vi "Target3.vi"() -> ()   [LabVIEW 2025]
uses:
  <vilib>/Platform/TimedLoop/XDataNode/timing_clust.ctl
  <vilib>/Platform/TimedLoop/XDataNode/nitl_modes.ctl
  <vilib>/Platform/TimedLoop/XDataNode/wakeup.ctl
  <vilib>/eio/utilities/niEioResolveVilibRelativePath.vi
  <vilib>/rvi/interface/RandomDataEmulation/niFpgaRandomDataHandleErrors.vi
  <vilib>/rvi/Emulation/niFpgaSctlEmulationGetInTimedLoop.vi
  <vilib>/rvi/Emulation/niFpgaEmulationReportErrorSimple.vi
  <vilib>/rvi/Emulation/niFpgaGetClockAttributes.vi
  <vilib>/rvi/Emulation/niFpgaCriticalErrorInLSC.vi
  <vilib>/rvi/linearAlgebra/MatrixMultiply/simVIs/SubVI/nifxpla_MatrixMultiply_SimMatrixSizes.vi
  <vilib>/rvi/linearAlgebra/MatrixMultiply/simVIs/SubVI/nifxpla_MatrixMultiply_Sim4WireAdapterVector.vi
  <vilib>/rvi/linearAlgebra/MatrixMultiply/simVIs/SubVI/nifxpla_MatrixMultiply_SimFrameHandShake.vi
  <vilib>/rvi/linearAlgebra/MatrixMultiply/simVIs/SubVI/nifxpla_MatrixMultiply_SimVectorDataBuffer.vi
  <vilib>/rvi/linearAlgebra/MatrixMultiply/simVIs/SubVI/nifxpla_MatrixMultiply_SimNestedIndex.vi
  <vilib>/rvi/ClientSDK/Core/DevComputerLib/Private/Multiply(dfxp64).vi
  <vilib>/rvi/ClientSDK/Core/DevComputerLib/Private/Dfxp128ToDfxp256.vi
  <vilib>/rvi/ClientSDK/Core/DevComputerLib/Private/Add(dfxp256).vi
  <vilib>/rvi/ClientSDK/Core/DevComputerLib/Private/Subtract(dfxp256).vi
  <vilib>/rvi/ClientSDK/Core/DevComputerLib/Private/ToDfxp64(dfxp256).vi
  <vilib>/rvi/DataTransferAndStorage/Container/XNode/niFpgaContainer.xnode
  <vilib>/rvi/interface/RandomDataEmulation/nirviRandomDataFpgaReadWriteTemplate.vi
  <vilib>/platform/TimedLoop/XDataNode/XDataNode.xnode
  <vilib>/rvi/linearAlgebra/MatrixMultiply/XNode/nifxpla_MatrixMultiply.xnode
  <vilib>/rvi/linearAlgebra/MatrixMultiply/simVIs/nifxpla_MatrixMultiply_SimTemplateEinEout.vi
  <vilib>/rvi/linearAlgebra/MatrixMultiply/simVIs/nifxpla_MatrixMultiply_SimTemplateEinVout.vi
  <vilib>/rvi/linearAlgebra/MatrixMultiply/simVIs/nifxpla_MatrixMultiply_SimTemplateVinEout.vi
  <vilib>/rvi/linearAlgebra/MatrixMultiply/simVIs/nifxpla_MatrixMultiply_SimTemplateVinVout.vi
  <vilib>/Platform/TimedLoop/XDataNode/XDNodeRunTimeDep.lvlib
panel:
  out "operation overflow":bool
  out "Array 4":fxp<+/-,32,16>[](array[numeric])
  out "Array 5":fxp<+/-,32,16>[](array[numeric])
  out "Array 2":bool[](array[boolean])
  out "Array":bool[](array[boolean])
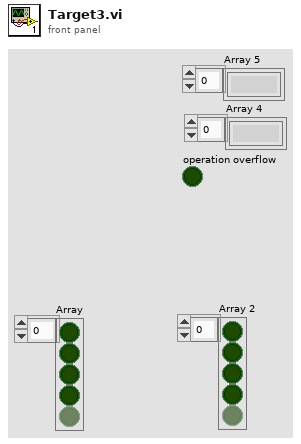
[diagram p1: front panel]
types:
  T1 = typedef "XDNodeRunTimeDep.lvlib/timing_clust.ctl" = cluster{"Expected End [f-1]":u64, "Actual End [f-1]":u64, "Finished Late? [f-1]":bool, "Expected End [i-1]":u64, "Actual End [i-1]":u64, "Finished Late? [i-1]":bool, "Expected Start [i]":u64, "Actual Start [i]":u64, "Expected Start [f]":u64, "Actual Start [f]":u64, "Source Name":string, "Structure Name":string, "Period":i64, "Deadline":i64, "Offset":i64, "Start":i64, "Priority":i32, "Timeout":i32, "Mode":T2, "Wakeup Reason":T3, "Error":errorcluster, "Source Type":string, "Secondary Source Type":string, "Global End Time":u64, "Global Start Time":u64, "Frame Duration":u64, "Iteration Duration":u64, "Assigned CPU":i32, "I/O Scan Engine Mode":u32}
  T2 = typedef "XDNodeRunTimeDep.lvlib/nitl_modes.ctl" = enum32{"No Change", "Process missed periods, maintain original phase", "Discard missed periods, maintain original phase", "Process missed periods, ignore original phase", "Discard missed periods, ignore original phase"}
  T3 = typedef "XDNodeRunTimeDep.lvlib/wakeup.ctl" = enum32{"Normal", "Aborted", "Asynchronous wakeup", "Timing source error", "Timed loop error", "Timeout"}
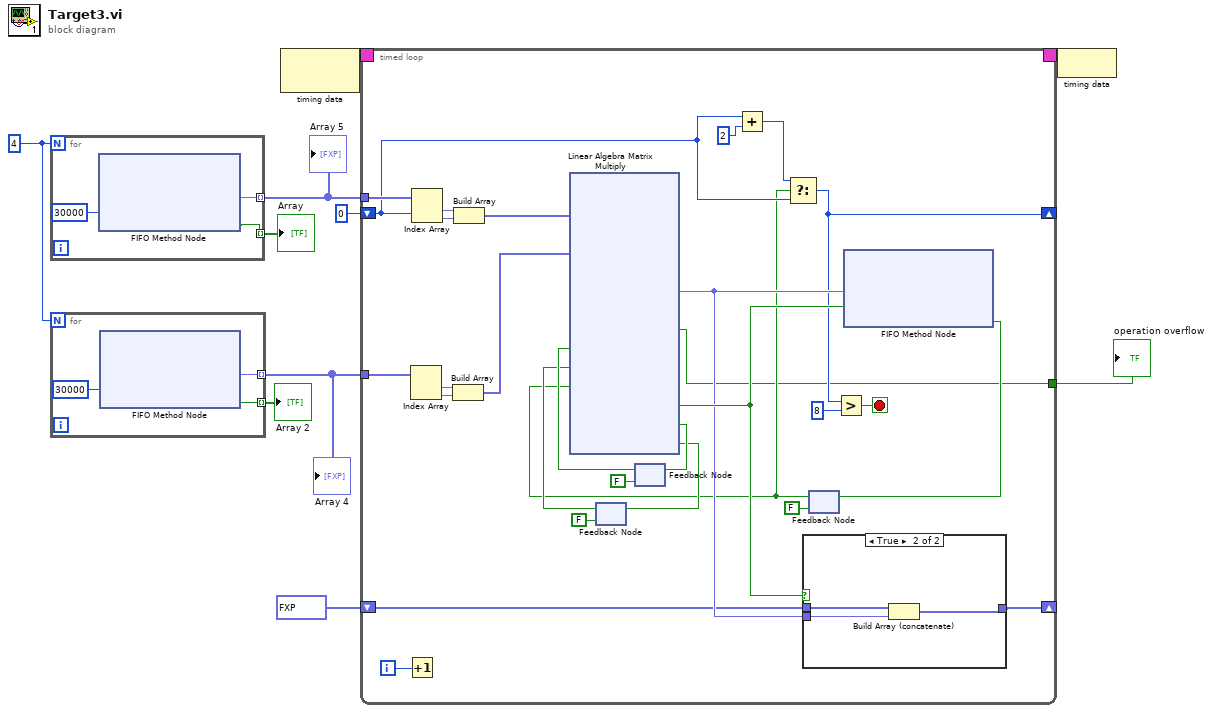
[diagram p0: block diagram]
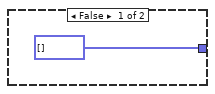
[diagram p2: hidden frame]
diagram:
  w5 = 4
  n1 = for {
    N: w5 -> [_]
    tunnel: [w13] -> w8 mode=indexing
    tunnel: [w11] -> w3 mode=indexing
    n2 = xnode ("FIFO Method Node")("Timeout"=30000) -> ("Element"=w13:fxp<+/-,32,16>, "Timed Out?"=w11:bool)  [unwired: 1 in, 1 out]
  }
  "Array" <- w3
  "Array 5" <- w8
  n3 = for {
    N: w5 -> [_]
    tunnel: [w16] -> w7 mode=indexing
    tunnel: [w14] -> w2 mode=indexing
    n4 = xnode ("FIFO Method Node")("Timeout"=30000) -> ("Element"=w16:fxp<+/-,32,16>, "Timed Out?"=w14:bool)  [unwired: 1 in, 1 out]
  }
  "Array 2" <- w2
  "Array 4" <- w7
  n5 = node-c288() -> (w10:T1)  [unwired: 1 in]
  n6 = timed-loop {
    timing: w10 -> [_]
    timing-out: [_] -> w9
    tunnel: w8 -> [w45]
    tunnel: w7 -> [w39]
    shift-right: [w20] -> _
    shift-left: 0 -> [w24]
    shift-right: [w29] -> _
    shift-left: fxp<+/-,64,35>[] [0.0, 0.0] ("cr") -> [w30]
    tunnel: [w17] -> w1
    i -> [w34]
    stop <- w21 stop-if-true
    n7 = Increment(x=w34) -> ()  [unwired: 1 out]
    n8 = Index Array(array=w39) -> (element #1=w41:fxp<+/-,32,16>, element #2=w40:fxp<+/-,32,16>)  [unwired: 2 in]
    n9 = Index Array(array=w45, index #1=w24) -> (element #1=w44:fxp<+/-,32,16>, element #2=w43:fxp<+/-,32,16>)  [unwired: 1 in]
    n10 = Build Array(w41, w40) -> (w38:fxp<+/-,32,16>[])
    n11 = Build Array(w44, w43) -> (w42:fxp<+/-,32,16>[])
    n12 = feedback #1(FALSE ("ready for b")) -> (w33:bool)
    n13 = feedback #2(FALSE ("ready for a")) -> (w35:bool)
    n14 = Add(x=w24, y=2) -> (x+y=w23:i32)
    n15 = feedback #3(FALSE ("Ready for Input")) -> (w22:bool)
    n16 = xnode ("Linear Algebra Matrix Multiply")("ar"=w42, "br"=w38, "a valid"=w35, "b valid"=w33, "ready for output (T)"=w22) -> ("cr"=w31:fxp<+/-,32,16>, "operation overflow"=w17:bool, "output valid"=w32:bool, "ready for a"=w37:bool, "ready for b"=w36:bool)  [unwired: 2 in, 1 out]
    n17 = feedback-in #1(w36) -> ()
    n18 = feedback-in #2(w37) -> ()
    n19 = Select(t=w23, s=w22, f=w24) -> (s? t:f=w20:i32)
    n20 = case shown="True" w32 {
      tunnel: [fxp<+,1,1>[] [] w49] -> w29
      tunnel: w31 -> [_ w47]
      tunnel: w30 -> [_ w48]
      frame False {
      }
      frame True {
        n21 = Build Array (concatenate)(w48, w47) -> (w49:fxp<+/-,64,35>[])
      }
    }
    n22 = Greater?(x=w20, y=8) -> (0:w21:bool)
    n23 = xnode ("FIFO Method Node")("Element"=w31, "Input Valid"=w32) -> ("Ready for Input"=w27:bool)  [unwired: 1 in, 1 out]
    n24 = feedback-in #3(w27) -> ()
  }
  "operation overflow" <- w1
  n25 = node-c288(w9) -> ()
